vi "2 MissionHeadingGoodness.vi"(9 "Heading to Test":T1 format="%05.1f", 11 "CurrentMission":refnum<class "GenericMission.lvclass">) -> (0 "Pure Waypoint Goodness":dbl, 1 "Direction Change Goodness":dbl, 2 "No-Sail Goodness":dbl, 3 "Target Goodness":dbl, 4 "Pure Wind Goodness":dbl)   [LabVIEW 2011]
doc: "This VI simply takes in a heading to test, runs the necessary component goodness functions and outputs their \"goodness value\" for that heading."
uses:
  2 Typedefs/heading.ctl
  2 Classes/Missions/GenericMission/GenericMission.lvclass
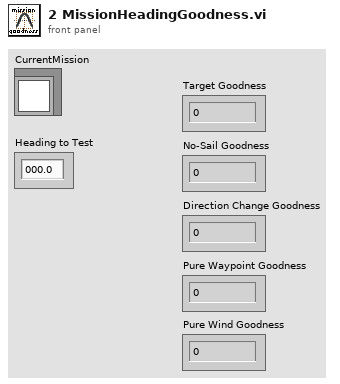
[diagram p1: front panel]
types:
  T1 = typedef "heading.ctl" = dbl
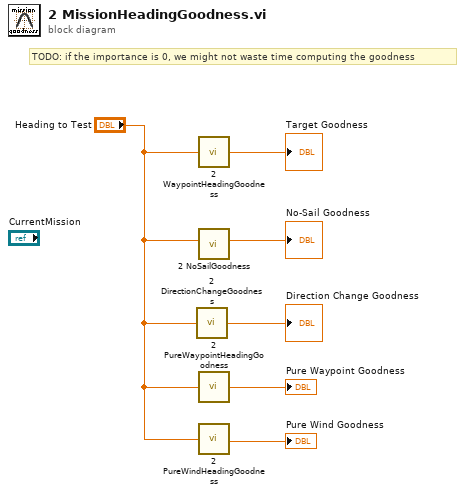
[diagram p0: block diagram]
diagram:
  # "TODO: if the importance is 0, we might not waste time computing the goodness"
  n1 = call "2 DirectionChangeGoodness.vi"("Test Heading"="Heading to Test") -> ("Goodness"=→"Direction Change Goodness":dbl)
  n2 = call "2 WaypointHeadingGoodness.vi"("Heading\nto Test"="Heading to Test") -> ("Goodness"=→"Target Goodness":dbl)  [unwired: 4 in]
  n3 = call "2 NoSailGoodness.vi"("Heading to Test"="Heading to Test") -> ("Goodness"=→"No-Sail Goodness":dbl)  [unwired: 10 in]
  n4 = call "2 PureWaypointHeadingGoodness.vi"("Heading to Test"="Heading to Test") -> ("Goodness"=→"Pure Waypoint Goodness":dbl)  [unwired: 4 in]
  n5 = call "2 PureWindHeadingGoodness.vi"("Heading\nto Test"="Heading to Test") -> ("Goodness"=→"Pure Wind Goodness":dbl)  [unwired: 4 in]
